vi "read_json_example.vi"() -> ()   [LabVIEW 2015]
panel:
  out "value 2":i32
  out "error out 4":errorcluster
  out "value 3":string
  out "error out 3":errorcluster
  out "nstims 2":i32
  out "error out 2":errorcluster
  out "value":string
  out "error out":errorcluster
  out "text":string
  in  "Path":path
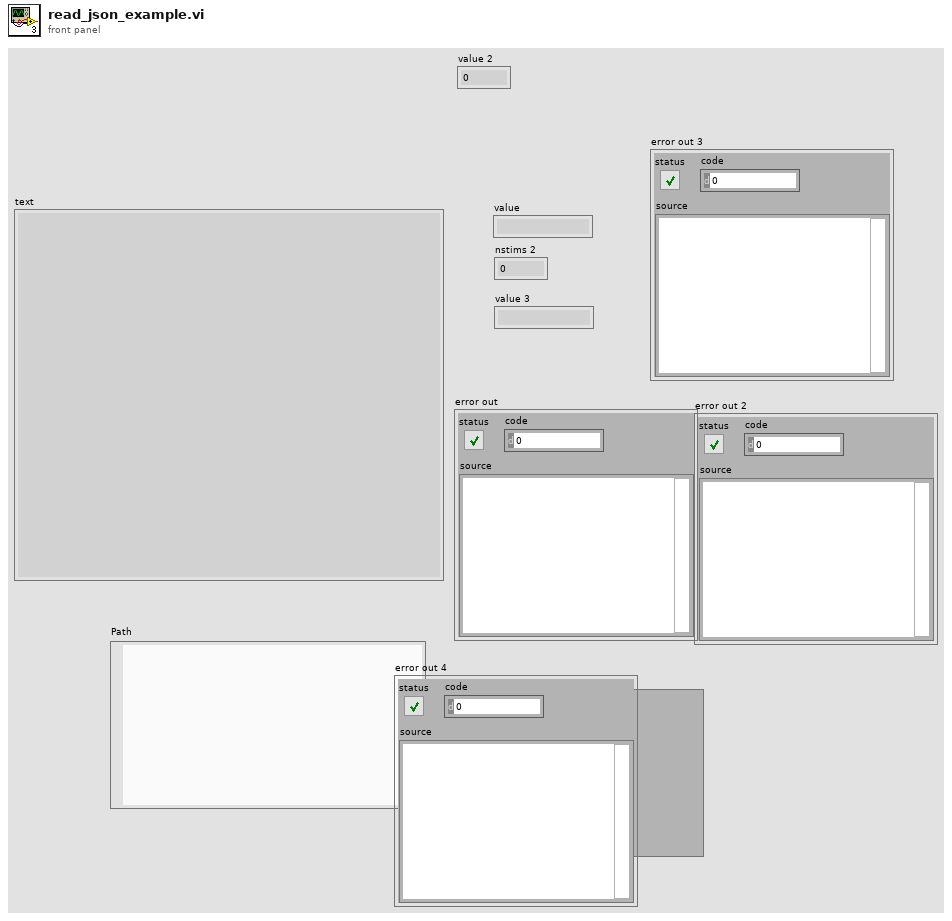
[diagram p1: front panel]
types:
  T1 = enum16{"open", "replace", "create", "open or create", "replace or create", "replace or create with confirmation"}
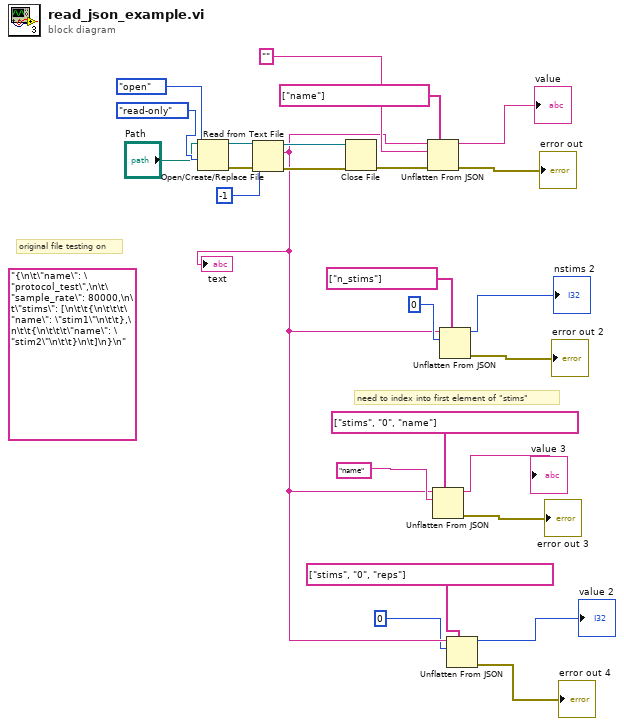
[diagram p0: block diagram]
diagram:
  (unwired) "{\n\t\"name\": \"protocol_test\",\n\t\"sample_rate\": 80000,\n\t\"stims\": [\n\t\t{\n\t\t\t\"name\": \"stim1\"\n\t\t},\n\t\t{\n\t\t\t\"name\": \"stim2\"\n\t\t}\n\t]\n}\n"
  # "need to index into first element of \"stims\""
  # "original file testing on"
  n1 = Open/Create/Replace File(file path (use dialog)="Path", operation (0:open)=T1."open", access (0:read/write)=enum16{"read/write", "read-only", "write-only"}."read-only") -> (refnum out=w23:refnum<file>, error out=w22:errorcluster)  [unwired: 3 in, 1 out]
  n2 = Read from Text File(file (use dialog)=w23, count=-1, error in=w22) -> (refnum out=w25:refnum<file>, text=w4:string, error out=w24:errorcluster)  [unwired: 1 in, 1 out]
  "text" <- w4
  n3 = Close File(refnum=w25, error in=w24) -> (error out=w19:errorcluster)  [unwired: 1 out]
  n4 = Unflatten From JSON(path=string[] ["name"], JSON string=w4, type and defaults="", error in (no error)=w19) -> (value=→"value":string, error out=→"error out":errorcluster)  [unwired: 3 in]
  n5 = Unflatten From JSON(path=string[] ["stims", "0", "name"], JSON string=w4, type and defaults="name") -> (value=→"value 3":string, error out=→"error out 3":errorcluster)  [unwired: 4 in]
  n6 = Unflatten From JSON(path=string[] ["n_stims"], JSON string=w4, type and defaults=0) -> (value=→"nstims 2":i32, error out=→"error out 2":errorcluster)  [unwired: 4 in]
  n7 = Unflatten From JSON(path=string[] ["stims", "0", "reps"], JSON string=w4, type and defaults=0) -> (value=→"value 2":i32, error out=→"error out 4":errorcluster)  [unwired: 4 in]
